vi "Trim String Whitespace.vi"(7 "Strip Whitespace? [T]":bool=TRUE, 8 "error in (no error)":errorcluster, 10 "String":string, 11 "Registry Object":refnum<class "Carya Config.lvclass">) -> (0 "error out":errorcluster, 2 "Trimmed string":string, 3 "Registry Object":refnum<class "Carya Config.lvclass">)   [LabVIEW 2013, in "Carya Config.lvclass"]
doc: "Copyright 2018, Carya Automatisering, Wiebe Walstra."
uses:
  Carya Config.lvclass
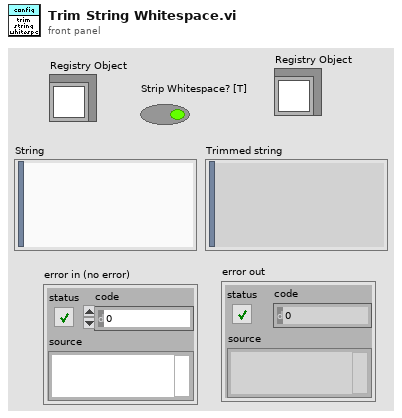
[diagram p1: front panel]
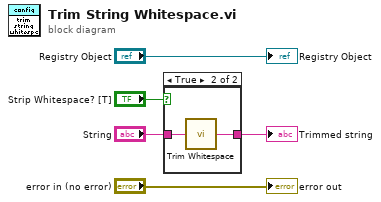
[diagram p0: block diagram]
diagram:
  n1 = case shown="True" "Strip Whitespace? [T]" {
    tunnel: [w6 w8] -> w3
    tunnel: "String" -> [w6 w7]
    frame False {
    }
    frame True {
      n2 = call <vilib>:"Trim Whitespace.vi"("string"=w7) -> ("trimmed string"=w8:string)  [unwired: 1 in]
    }
  }
  "Trimmed string" <- w3
  "Registry Object" <- "Registry Object"
  "error out" <- "error in (no error)"
